vi "LibXML_GetNodeElementType.vi"(8 "error in":errorcluster, 11 "node":u32) -> (0 "error out":errorcluster, 2 "element type (integer)":i32, 3 "element type":T1(ring))   [LabVIEW 2019, in "Tools.lvlib" / "LibXML.lvlib"]
doc: "Gets the node type of node input."
uses:
  LibXML.lvlib
  dll/lXMLwrap.dll
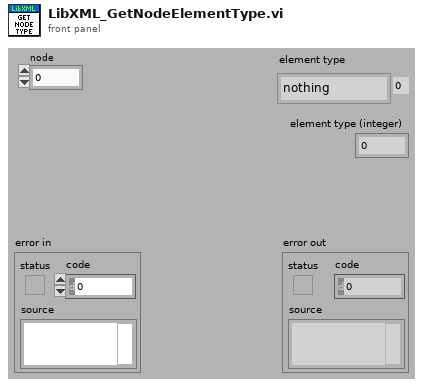
[diagram p1: front panel]
types:
  T1 = enum16{"nothing", "element", "attribute", "text", "cdata", "5 or more"}
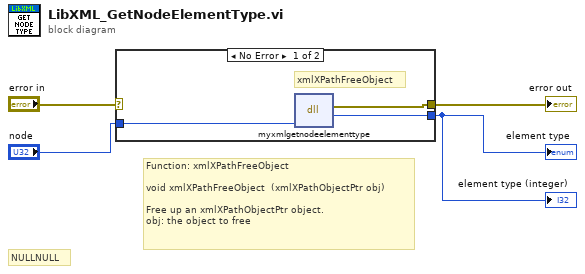
[diagram p0: block diagram]
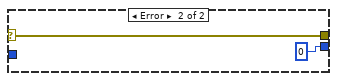
[diagram p2: hidden frame]
diagram:
  # "NULLNULL"
  # "Function: xmlXPathFreeObject\n\nvoid\txmlXPathFreeObject\t\t(xmlXPathObjectPtr obj)\n\nFree up an xmlXPathObjectPtr object.\nobj:\tthe object to free"
  n1 = case shown="No Error" "error in" {
    selector: "error in" -> [_ w9]
    tunnel: [w5 w9] -> w3
    tunnel: "node" -> [w7 _]
    tunnel: [w6 0] -> w1
    frame No Error {
      # "xmlXPathFreeObject"
      n2 = dll-call lib="C:/Projects/_Prywatne/MyCIT/Framework/Tools/XML/LibXML/dll/lXMLwrap.dll" fn="myxmlgetnodeelementtype"("XPathObj"=w7) -> (error out=w5:errorcluster, "return type"=w6:i32)  [unwired: 4 in, 1 out]
    }
    frame Error {
    }
  }
  "error out" <- w3
  "element type (integer)" <- w1
  "element type" <- w1
